vi "get display name.vi"(8 "error in":errorcluster, 11 "reset to origin in":refnum<class "reset to origin.lvclass">) -> (0 "error out":errorcluster, 2 "class name":string, 3 "reset to origin out":refnum<class "reset to origin.lvclass">)   [LabVIEW 2013, in "reset to origin.lvclass"]
uses:
  reset to origin.lvclass
  VI modification.lvclass
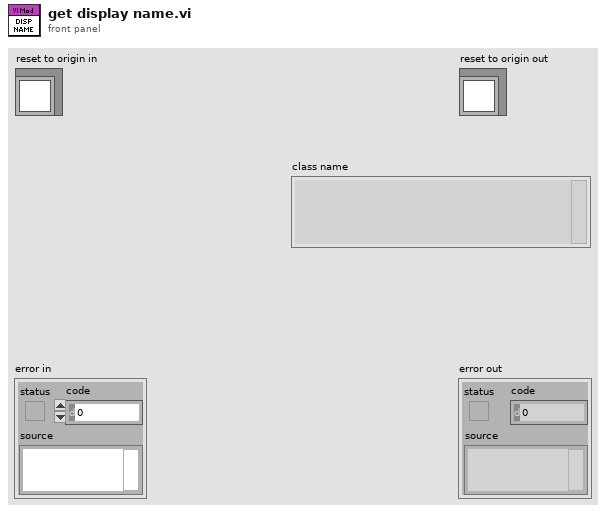
[diagram p1: front panel]
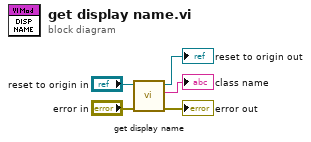
[diagram p0: block diagram]
diagram:
  n1 = call-parent "get display name.vi"("error in"="error in", "VI modification in"="reset to origin in") -> ("error out"=→"error out":errorcluster, "class name"=→"class name":string, "VI modification out"=→"reset to origin out":refnum<class "reset to origin.lvclass">)  [unwired: 7 in]
